vi "New_Giris (SubVI).vi"() -> (0 "Type 2":string, 1 "OKTO":bool, 2 "Username 2":string)   [LabVIEW 2009]
uses:
  <vilib>/Utility/file.llb/Read From Spreadsheet File (string).vi
panel:
  in  "Encode/Decode":bool
  in  "Magnitude of Shift":u8=22
  out "Type":string
  in  "Şifre":string caption="Password"
  in  "Kullanıcı Adı":string caption="Username"
  in  "OK":bool caption="OK2"
  in  "Cancel":bool
  # "Lütfen Uygun Kullanıcı Adı ve Şifre Giriniz"
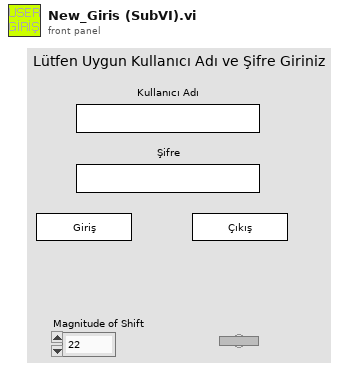
[diagram p1: front panel]
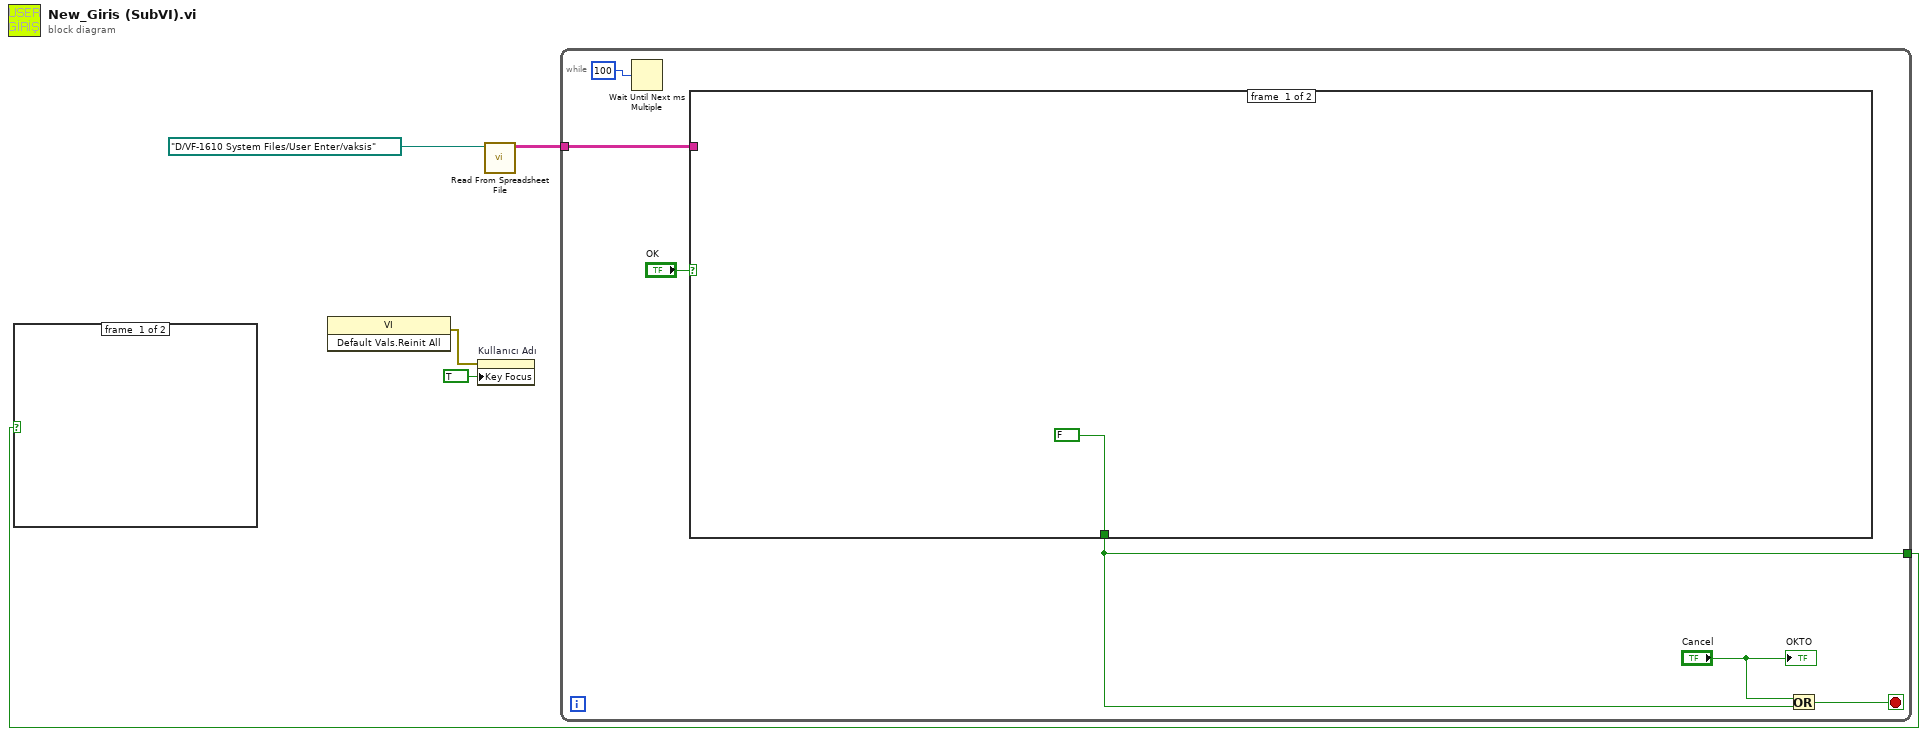
[diagram p0: block diagram]
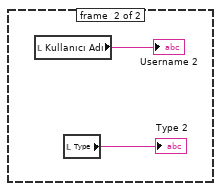
[diagram p2: hidden frame]
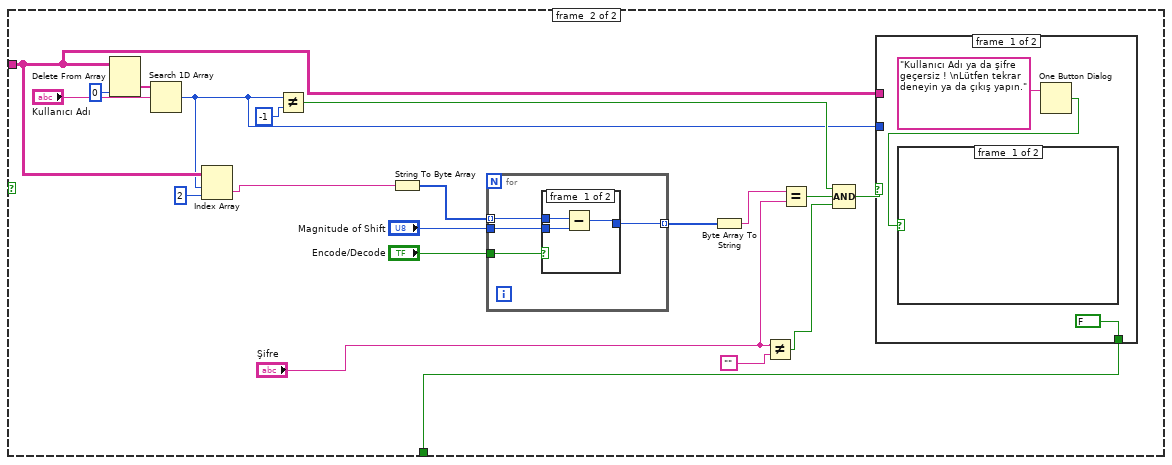
[diagram p3: hidden frame]
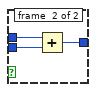
[diagram p4: hidden frame]
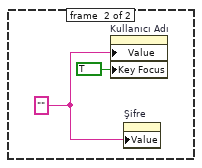
[diagram p5: hidden frame]
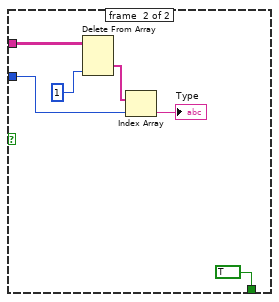
[diagram p6: hidden frame]
diagram:
  n1 = invoke class="VI" method="Default Vals.Reinit All"() -> (error out=w2:errorcluster)  [unwired: 3 in, 2 out]
  n2 = property on="Kullanıcı Adı" class="Str"(error in=w2, "Key Focus"=TRUE) -> ()  [unwired: 1 in, 2 out]
  n3 = call-poly <vilib>:"Read From Spreadsheet File.vi"("file path (dialog if empty)"=path "D:/VF-1610 System Files/User Enter/vaksis" ("Path")) -> ("all rows"=w4:string[][])  [unwired: 6 in, 4 out]
  n4 = while {
    tunnel: w4 -> [w11]
    tunnel: [w8] -> w3
    stop <- w10 stop-if-true
    n5 = Wait Until Next ms Multiple(millisecond multiple=100) -> ()  [unwired: 1 out]
    n6 = case shown="True" "OK" {
      tunnel: w11 -> [_ w24]
      tunnel: [FALSE w25] -> w8
      frame #0 {
      }
      frame #1 {
        n7 = Delete From Array(array=w24, index (col)=0 ("disabled index (col)")) -> (deleted portion=w30:string[])  [unwired: 2 in, 1 out]
        n8 = Search 1D Array(1D array=w30, element="Kullanıcı Adı") -> (index of element=w22:i32)  [unwired: 1 in]
        n9 = Index Array(array=w24, index (row)=w22, index (col)=2 ("disabled index (col)")) -> (element=w17:string)
        n10 = Not Equal?(x=w22, y=-1) -> (x != y?=w28:bool)
        n11 = String To Byte Array(string=w17) -> (unsigned byte array=w18:u8[])
        n12 = for {
          tunnel: w18 -> [w36] mode=indexing
          tunnel: "Magnitude of Shift" -> [w35]
          tunnel: [w34] -> w20 mode=indexing
          tunnel: "Encode/Decode" -> [w33]
          n13 = case shown="False" w33 {
            tunnel: w36 -> [w38 w42]
            tunnel: w35 -> [w39 w41]
            tunnel: [w37 w40] -> w34
            frame #0 {
              n14 = Subtract(x=w38, y=w39) -> (x-y=w37:u8)
            }
            frame #1 {
              n15 = Add(x=w42, y=w41) -> (x+y=w40:u8)
            }
          }
        }
        n16 = Byte Array To String(unsigned byte array=w20) -> (string=w16:string)
        n17 = Not Equal?(x="Şifre", y="") -> (x != y?=w13:bool)
        n18 = Equal?(x=w16, y="Şifre") -> (x = y?=w27:bool)
        n19 = Compound Arithmetic op=AND(w28, w27, w13) -> (w26:bool)
        n20 = case shown="False" w26 {
          tunnel: [FALSE TRUE] -> w25
          tunnel: w22 -> [_ w49]
          tunnel: w24 -> [_ w51]
          frame #0 {
            n21 = One Button Dialog(message="Kullanıcı Adı ya da şifre geçersiz ! \nLütfen tekrar deneyin ya da çıkış yapın.") -> (true=w43:bool)  [unwired: 1 in]
            n22 = case shown="True" w43 {
              frame #0 {
              }
              frame #1 {
                w47 = "" ("Password")
                n23 = property on="Kullanıcı Adı" class="Str"("Value"=w47, "Key Focus"=TRUE) -> ()  [unwired: 2 in, 2 out]
                n24 = property on="Şifre" class="Str"("Value"=w47) -> ()  [unwired: 2 in, 2 out]
              }
            }
          }
          frame #1 {
            n25 = Delete From Array(array=w51, index (col)=1 ("disabled index (col)")) -> (deleted portion=w50:string[])  [unwired: 2 in, 1 out]
            n26 = Index Array(array=w50, index=w49) -> (element=→"Type":string)
          }
        }
      }
    }
    n27 = Or(x="Cancel", y=w8) -> (x .or. y?=w10:bool)
    "OKTO" <- "Cancel"
  }
  n28 = case shown="True" w3 {
    frame #0 {
    }
    frame #1 {
      n29 = local read "Kullanıcı Adı"() -> (→"Username 2":string)
      n30 = local read "Type"() -> (→"Type 2":string)
    }
  }
